vi "Get VI Metadata.vi"(8 "error in":errorcluster, 11 "VI ref in":refnum<vi>) -> (0 "error out":errorcluster, 2 "Metadata":T1, 3 "VI ref out":refnum<vi>)   [LabVIEW 2019]
doc: "Get information about the VI and creates an HTML content to be used in the main viewer."
uses:
  Typedefs/VI Metadata.ctl
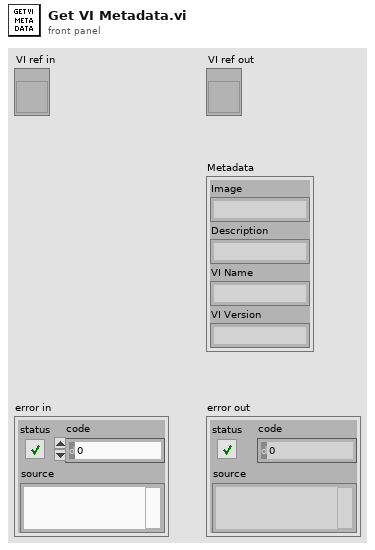
[diagram p1: front panel]
types:
  T1 = typedef "VI Metadata.ctl" = cluster{"Image":string, "Description":string, "VI Name":string, "VI Version":string}
  T2 = enum32{"invalid VI type", "Standard VI", "Control VI", "Global VI", "Polymorphic VI", "Configuration VI", "SubSystem", "Facade VI", "Method VI", "Statechart Diagram VI"}
  T3 = typedef "imagedata.ctl" = cluster{"image type":i32, "image depth":i32, "image":u8[], "mask":u8[], "colors":u32[], "Rectangle":cluster{"left":i16, "top":i16, "right":i16, "bottom":i16}}
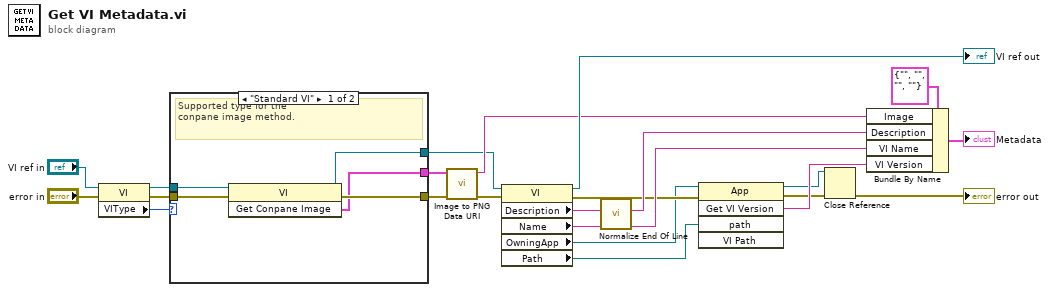
[diagram p0: block diagram]
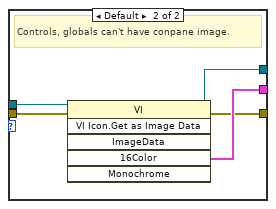
[diagram p2: hidden frame]
diagram:
  n1 = property class="VI"(reference="VI ref in", error in="error in") -> (reference out=w20:refnum<vi>, error out=w22:errorcluster, "VIType"=w21:T2)
  n2 = case shown="\"Standard VI\"" w21 {
    tunnel: w22 -> [w28 w29]
    tunnel: [w26 w30] -> w16
    tunnel: w20 -> [w27 w32]
    tunnel: [w25 w31] -> w8
    tunnel: [w24 w33] -> w18
    frame "Standard VI" {
      # "Supported type for the \nconpane image method."
      n3 = invoke class="VI" method="Get Conpane Image"(reference=w27, error in=w28) -> (reference out=w25:refnum<vi>, error out=w26:errorcluster, "Get Conpane Image"=w24:T3)  [unwired: 1 in]
    }
    frame Default {
      # "Controls, globals can't have conpane image."
      n4 = invoke class="VI" method="VI Icon.Get as Image Data"(reference=w32, error in=w29) -> (reference out=w31:refnum<vi>, error out=w30:errorcluster, "16Color"=w33:T3)  [unwired: 4 in, 3 out]
    }
  }
  n5 = call "Image to PNG Data URI.vi"("error in (no error)"=w16, "Image data"=w18) -> ("error out"=w15:errorcluster, "Base64 encoded"=w17:string)  [unwired: 7 in, 1 out]
  n6 = property class="VI"(reference=w8, error in=w15) -> (reference out=→"VI ref out":refnum<vi>, error out=w7:errorcluster, "Description"=w12:string, "Name"=w13:string, "OwningApp"=w6:refnum<vi>, "Path"=w5:path)
  n7 = call <vilib>:"Normalize End Of Line.vi"("string in"=w12) -> ("string out"=w11:string)  [unwired: 7 in]
  n8 = invoke class="App" method="Get VI Version"(reference=w6, error in=w7, "path"=w5) -> (reference out=w2:refnum<vi>, error out=w3:errorcluster, "GetVIVers"=w4:string)  [unwired: 2 in, 2 out]
  n9 = Close Reference(reference=w2, error in (no error)=w3) -> (error out=→"error out":errorcluster)
  n10 = Bundle By Name(cluster=T1 {"Image"="", "Description"="", "VI Name"="", "VI Version"=""} ("Metadata"), "Image"=w17, "Description"=w11, "VI Name"=w13, "VI Version"=w4) -> (→"Metadata":T1)
